vi "PathMessageLibrary.vi"() -> (2 "Path":path)   [LabVIEW 2017, in "MessageGen.lvlib"]
uses:
  <vilib>/addons/InsightCM/MessageBus/CodeGen/MessageGen.lvlib
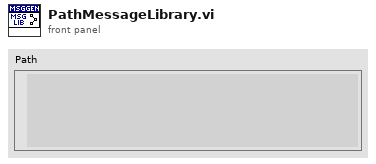
[diagram p1: front panel]
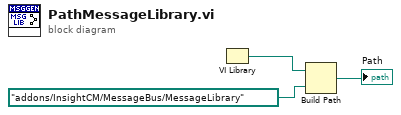
[diagram p0: block diagram]
diagram:
  n1 = VI Library() -> (path=w3:path)
  n2 = Build Path(base path=w3, name or relative path=path "addons/InsightCM/MessageBus/MessageLibrary") -> (appended path=→"Path":path)
